vi "Create.vi"(8 "error in (no error)":errorcluster, 11 "Server":string) -> (0 "error out":errorcluster, 3 "LDAP Authentication out":refnum<class "LDAP Authentication.lvclass">)   [LabVIEW 2016, in "LDAP Authentication.lvclass"]
uses:
  LDAP Authentication.lvclass
  LDAP Authentication.lvclass/LDAP Authentication.ctl
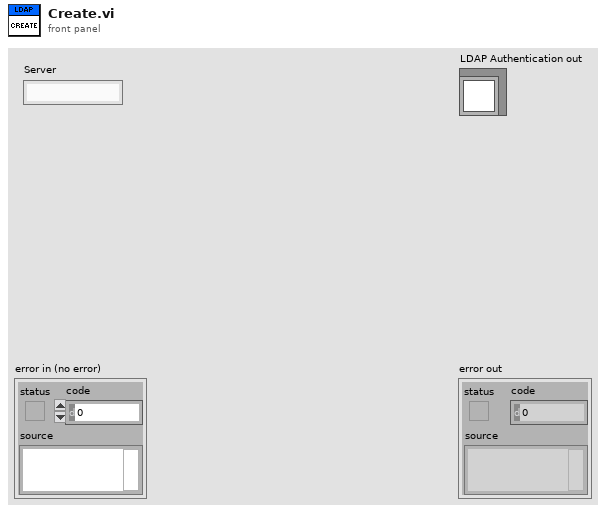
[diagram p1: front panel]
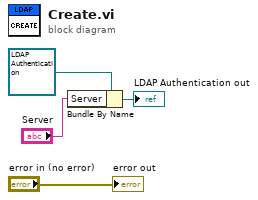
[diagram p0: block diagram]
diagram:
  n1 = Bundle By Name(cluster=refnum<class "LDAP Authentication.lvclass"> refnum ("LDAP Authentication out"), "Server"="Server") -> (→"LDAP Authentication out":refnum<class "LDAP Authentication.lvclass">)
  "error out" <- "error in (no error)"
